vi "TCPPacket Read Body.vi"(8 "error in (no error)":errorcluster, 10 "Data":u8[](array[numeric]), 11 "JSONPacket in":refnum<class "JSONPacket.lvclass">) -> (0 "error out":errorcluster, 3 "JSONPacket out":refnum<class "JSONPacket.lvclass">)   [LabVIEW 2019, in "JSONPacket.lvclass"]
uses:
  JSONPacket.lvclass
  JSONPacket.lvclass/JSONPacket.ctl
  <vilib>/addons/Tools/Unicode/UTF8 Tools.lvlib
  c414942a-5d98-42c7-a9c9-eaca4a0c31ce.vi
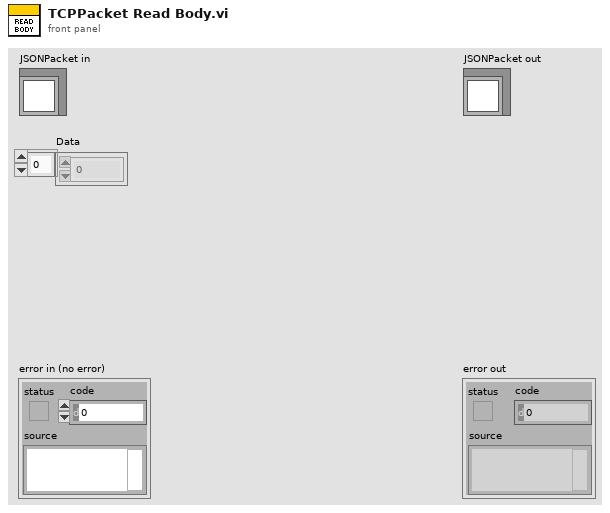
[diagram p1: front panel]
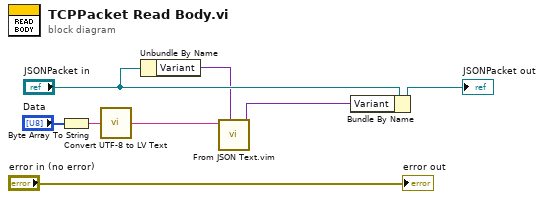
[diagram p0: block diagram]
diagram:
  n1 = Byte Array To String(unsigned byte array="Data") -> (string=w6:string)
  n2 = call <vilib>:"Convert UTF-8 to LV Text.vi"("UTF-8 Text"=w6) -> ("LV Text"=w3:string)  [unwired: 13 in, 1 out]
  n3 = Unbundle By Name("JSONPacket in") -> ("Variant"=w2:variant)
  n4 = call "From JSON Text.vim"("Data Type and Default Value"=w2, "JSON"=w3) -> ("Data out"=w1:variant)  [unwired: 8 in, 1 out]
  n5 = Bundle By Name(cluster="JSONPacket in", "Variant"=w1) -> (→"JSONPacket out":refnum<class "JSONPacket.lvclass">)
  "error out" <- "error in (no error)"
